vi "Configure Pulse.vi"(6 "Pulse Transition Time (2.00E-8 s)":dbl=2e-08 min=5e-09 max=0.001 format="%.2e", 8 "error in (no error)":errorcluster, 9 "Pulse Width (1.0 sec)":dbl=1.0 min=8e-09 max=2000.0 format="%.4f", 10 "Pulse Period (2.0 sec)":dbl=2.0 format="%.4g", 11 "VISA resource name":refnum<visa-resource-name>) -> (0 "error out":errorcluster, 3 "VISA resource name out":refnum<visa-resource-name>)   [LabVIEW 2017, in "Agilent 33XXX Series.lvlib"]
doc: "Sets the parameters for pulse waveforms.\n\nNote:\n(1) This VI is only used with the Agilent 33210A, 33220A and 33250A."
uses:
  Agilent 33XXX Series.lvlib
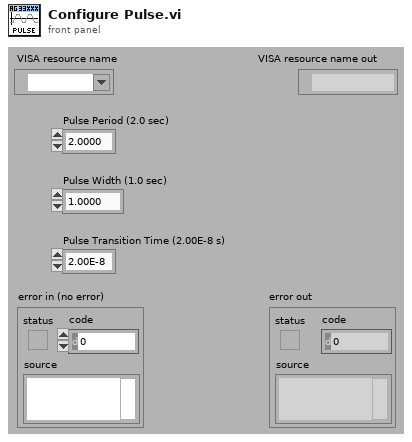
[diagram p1: front panel]
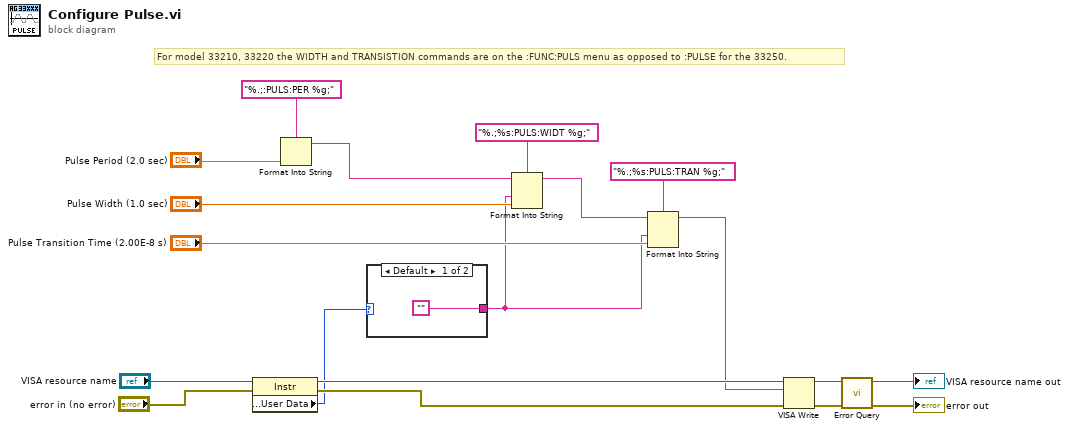
[diagram p0: block diagram]
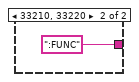
[diagram p2: hidden frame]
diagram:
  # "For model 33210, 33220 the WIDTH and TRANSISTION commands are on the :FUNC:PULS menu as opposed to :PULSE for the 33250."
  n1 = property class="Instr"(reference="VISA resource name", error in="error in (no error)") -> (reference out=w18:refnum<visa-resource-name>, error out=w19:errorcluster, "General Settings:User Data"=w1:u32)
  n2 = Format Into String(format string="%.;:PULS:PER %g;", "Pulse Period (2.0 sec)") -> (resulting string=w9:string)  [unwired: 2 in, 1 out]
  n3 = case shown="Default" w1 {
    tunnel: ["" ":FUNC"] -> w2
    frame Default {
    }
    frame 33210, 33220 {
    }
  }
  n4 = Format Into String(format string="%.;%s:PULS:WIDT %g;", initial string=w9, w2, "Pulse Width (1.0 sec)") -> (resulting string=w13:string)  [unwired: 1 in, 1 out]
  n5 = Format Into String(format string="%.;%s:PULS:TRAN %g;", initial string=w13, w2, "Pulse Transition Time (2.00E-8 s)") -> (resulting string=w7:string)  [unwired: 1 in, 1 out]
  n6 = VISA Write(VISA resource name=w18, write buffer=w7, error in (no error)=w19) -> (VISA resource name out=w17:refnum<visa-resource-name>, error out=w16:errorcluster)  [unwired: 1 out]
  n7 = call "Error Query.vi"("error in (no error)"=w16, "VISA resource name"=w17) -> ("error out"=→"error out":errorcluster, "VISA resource name out"=→"VISA resource name out":refnum<visa-resource-name>)  [unwired: 6 in, 2 out]
